vi "RotApp_LoadConfig.vi"(11 "configuration file":path) -> ()   [LabVIEW 2012]
uses:
  <vilib>/Utility/config.llb/Read Key (Double).vi
  RotationProgram/Global/RotationGlobal.vi
  <vilib>/Utility/config.llb/Read Key (String).vi
  <vilib>/Utility/config.llb/Read Key (Path).vi
  <vilib>/Utility/config.llb/NI_LVConfig.lvlib
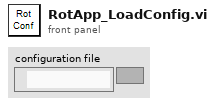
[diagram p1: front panel]
types:
  T1 = typedef "NI_LVConfig.lvlib/Config Data RefNum.ctl" = refnum<k1>
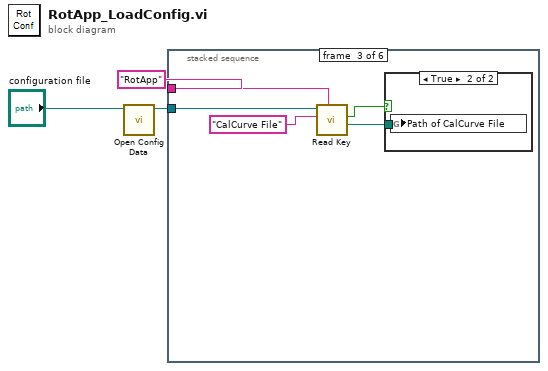
[diagram p0: block diagram]
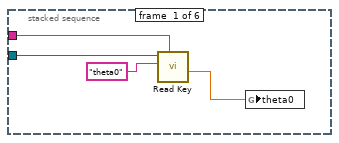
[diagram p2: hidden frame]
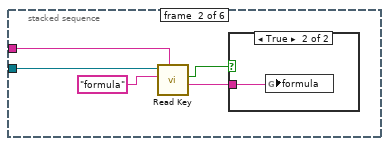
[diagram p3: hidden frame]
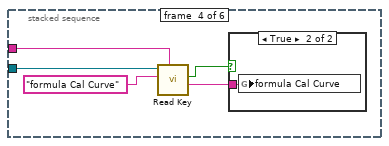
[diagram p6: hidden frame]
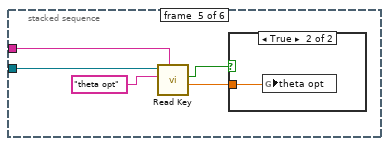
[diagram p8: hidden frame]
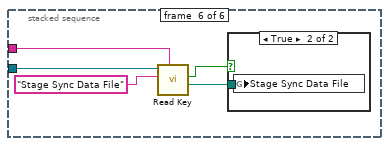
[diagram p10: hidden frame]
diagram:
  n1 = call <vilib>:"Open Config Data.vi"("configuration file path"="configuration file") -> ("refnum"=w2:T1)  [unwired: 8 in, 2 out]
  n2 = stacked-sequence {
    tunnel: w2 -> [w7 w12 w18 w24 w30 w36]
    tunnel: "RotApp" ("section") -> [w6 w11 w17 w23 w29 w35]
    frame #0 {
      n3 = call-poly <vilib>:"Read Key.vi"("section"=w6, "key"="theta0", "refnum"=w7) -> ("value"=w4:dbl)  [unwired: 5 in, 3 out]
      n4 = global write "RotationGlobal.vi" "theta0"(w4) -> ()
    }
    frame #1 {
      n5 = call-poly <vilib>:"Read Key.vi"("section"=w11, "key"="formula", "refnum"=w12) -> ("value"=w8:string, "found?"=w9:bool)  [unwired: 5 in, 2 out]
      n6 = case shown="True" w9 {
        tunnel: w8 -> [_ w13]
        frame False {
        }
        frame True {
          n7 = global write "RotationGlobal.vi" "formula"(w13) -> ()
        }
      }
    }
    frame #2 {
      n8 = call-poly <vilib>:"Read Key.vi"("section"=w17, "key"="CalCurve File", "refnum"=w18) -> ("value"=w14:path, "found?"=w15:bool)  [unwired: 5 in, 2 out]
      n9 = case shown="True" w15 {
        tunnel: w14 -> [_ w19]
        frame False {
        }
        frame True {
          n10 = global write "RotationGlobal.vi" "Path of CalCurve File"(w19) -> ()
        }
      }
    }
    frame #3 {
      n11 = call-poly <vilib>:"Read Key.vi"("section"=w23, "key"="formula Cal Curve", "refnum"=w24) -> ("value"=w20:string, "found?"=w21:bool)  [unwired: 5 in, 2 out]
      n12 = case shown="True" w21 {
        tunnel: w20 -> [_ w25]
        frame False {
        }
        frame True {
          n13 = global write "RotationGlobal.vi" "formula Cal Curve"(w25) -> ()
        }
      }
    }
    frame #4 {
      n14 = call-poly <vilib>:"Read Key.vi"("section"=w29, "key"="theta opt", "refnum"=w30) -> ("value"=w26:dbl, "found?"=w27:bool)  [unwired: 5 in, 2 out]
      n15 = case shown="True" w27 {
        tunnel: w26 -> [_ w31]
        frame False {
        }
        frame True {
          n16 = global write "RotationGlobal.vi" "theta opt"(w31) -> ()
        }
      }
    }
    frame #5 {
      n17 = call-poly <vilib>:"Read Key.vi"("section"=w35, "key"="Stage Sync Data File", "refnum"=w36) -> ("value"=w32:path, "found?"=w33:bool)  [unwired: 5 in, 2 out]
      n18 = case shown="True" w33 {
        tunnel: w32 -> [_ w37]
        frame False {
        }
        frame True {
          n19 = global write "RotationGlobal.vi" "Stage Sync Data File"(w37) -> ()
        }
      }
    }
  }
